vi "Halt all Commands.vi"(7 "error in (no error)":errorcluster, 10 "VISA in":refnum<visa-resource-name>) -> (0 "error out":errorcluster, 3 "VISA out":refnum<visa-resource-name>)   [LabVIEW 2018, in "ASI TG-1000.lvlib"]
doc: "Checks whether the motors are running; the equivalent of using the STATUS command."
uses:
  ASI TG-1000.lvlib
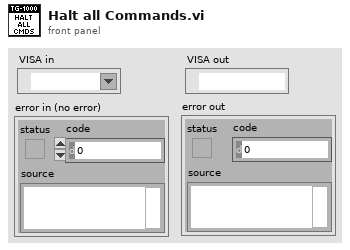
[diagram p1: front panel]
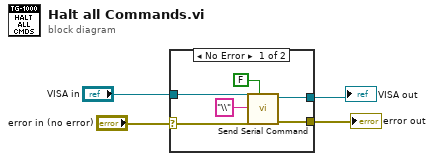
[diagram p0: block diagram]
diagram:
  n1 = case shown="No Error" "error in (no error)" {
    selector: "error in (no error)" -> [w6 w12]
    tunnel: "VISA in" -> [w10 w11]
    tunnel: [w9 w11] -> w3
    tunnel: [w8 w12] -> w2
    frame No Error {
      n2 = call "Send Serial Command.vi"("Listen for response (T)"=FALSE, "error in (no error)"=w6, "Command"="\\", "VISA in"=w10) -> ("error out"=w8:errorcluster, "VISA out"=w9:refnum<visa-resource-name>)  [unwired: 5 in, 1 out]
    }
    frame Error {
    }
  }
  "VISA out" <- w3
  "error out" <- w2
